vi "StartDebugClient.vi"(1 "target address":string="localhost", 2 "TCP port":u16=62001, 5 "error in (no error)":errorcluster) -> (19 "error out":errorcluster)   [LabVIEW 2017, in "G#RemoteProxy.lvclass"]
doc: "Starts the debug client process that makes it possible for debugger on the client host to debug objects on the remote target."
uses:
  G#RemoteProxy.lvclass
  G#Object/G#Object.lvclass
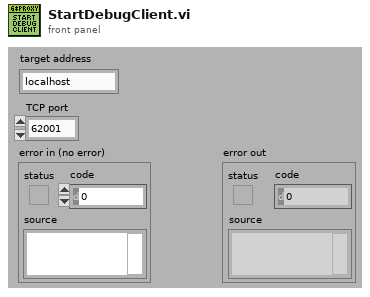
[diagram p1: front panel]
types:
  T1 = enum32{"Bad", "Idle", "Run top level", "Running"}
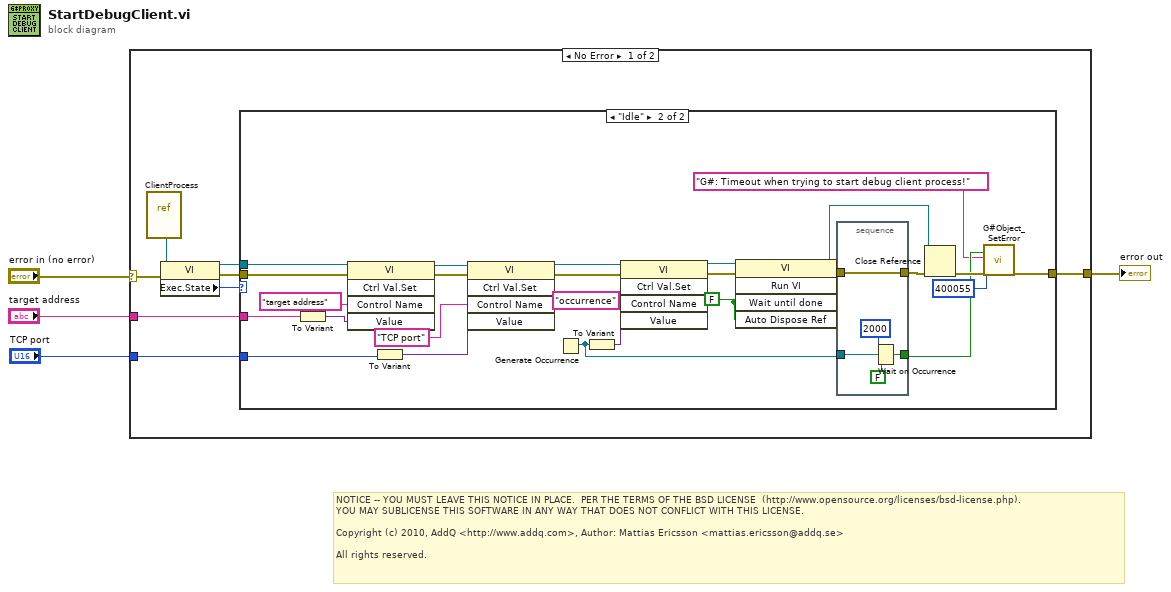
[diagram p0: block diagram]
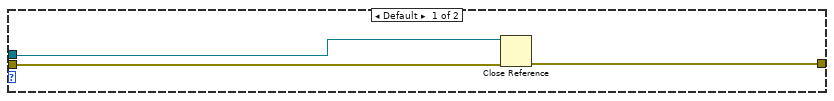
[diagram p2: hidden frame]
diagram:
  # "NOTICE -- YOU MUST LEAVE THIS NOTICE IN PLACE.  PER THE TERMS OF THE BSD LICENSE  (http://www.opensource.org/licenses/bsd-license.php).\nYOU MAY SUBLICENSE THIS SOFTWARE IN ANY WAY THAT DOES NOT CONFLICT WITH THIS LICENSE.\n\nCopyright (c) 2010, AddQ <http://www.addq.com>, Author: Mattias Ericsson <mattias.ericsson@addq.se>\n\nAll rights reserved."
  n1 = case shown="No Error" "error in (no error)" {
    selector: "error in (no error)" -> [w6 w47]
    tunnel: [w8 w47] -> w3
    tunnel: "target address" -> [w7 _]
    tunnel: "TCP port" -> [w5 _]
    frame No Error {
      n2 = vi-ref "ClientProcess.vi"() -> (w12:refnum<vi>)
      n3 = property class="VI"(reference=w12, error in=w6) -> (reference out=w9:refnum<vi>, error out=w10:errorcluster, "Exec.State"=w11:T1)
      n4 = case shown="\"Idle\"" w11 {
        tunnel: w10 -> [w15 w27]
        tunnel: w9 -> [w13 w26]
        tunnel: [w14 w31] -> w8
        tunnel: w7 -> [_ w23]
        tunnel: w5 -> [_ w17]
        frame Default {
          n5 = Close Reference(reference=w13, error in (no error)=w15) -> (error out=w14:errorcluster)
        }
        frame "Idle" {
          w37 = FALSE ("Wait Until Done")
          n6 = To Variant(anything=w23) -> (Variant=w24:variant)
          n7 = invoke class="VI" method="Ctrl Val.Set"(reference=w26, error in=w27, "Control Name"="target address", "Value"=w24) -> (reference out=w22:refnum<vi>, error out=w21:errorcluster)  [unwired: 1 in, 3 out]
          n8 = To Variant(anything=w17) -> (Variant=w16:variant)
          n9 = invoke class="VI" method="Ctrl Val.Set"(reference=w22, error in=w21, "Control Name"="TCP port", "Value"=w16) -> (reference out=w19:refnum<vi>, error out=w20:errorcluster)  [unwired: 1 in, 3 out]
          n10 = Generate Occurrence() -> (w35:refnum<k4>)
          n11 = To Variant(anything=w35) -> (Variant=w40:variant)
          n12 = invoke class="VI" method="Ctrl Val.Set"(reference=w19, error in=w20, "Control Name"="occurrence", "Value"=w40) -> (reference out=w38:refnum<vi>, error out=w39:errorcluster)  [unwired: 1 in, 3 out]
          n13 = invoke class="VI" method="Run VI"(reference=w38, error in=w39, "Wait until done"=w37, "Auto Dispose Ref"=w37) -> (reference out=w33:refnum<vi>, error out=w36:errorcluster)  [unwired: 1 in, 3 out]
          n14 = stacked-sequence {
            tunnel: w36 -> [w44]
            tunnel: w35 -> [w46]
            tunnel: [w44] -> w34
            tunnel: [w43] -> w30
            frame #0 {
              n15 = Wait on Occurrence(1:FALSE ("ignore previous (T)"), 2:w46, 3:2000 ("ms timeout (-1)")) -> (0:w43:bool)
            }
          }
          n16 = Close Reference(reference=w33, error in (no error)=w34) -> (error out=w32:errorcluster)
          n17 = call "G#Object_SetError.vi"("error (F)"=w30, "source"="G#: Timeout when trying to start debug client process!", "code"=400055, "error in (no error)"=w32) -> ("error out"=w31:errorcluster)  [unwired: 15 in]
        }
      }
    }
    frame Error {
    }
  }
  "error out" <- w3
